vi "Mixed.vi"() -> ()   [LabVIEW 2013]
uses:
  <vilib>/Analysis/4window.llb/windowTd.ctl
  <vilib>/Analysis/NI_AALPro.lvlib
  <vilib>/measure/maspectr.llb/Power Spectrum and PSD Export Mode.ctl
  <vilib>/measure/NI_MAPro.lvlib
  <vilib>/sound2/lvsound2.llb/Sound Output Set Volume (Single).vi
  <vilib>/measure/maspectr.llb/FFT Power Spectrum and PSD for 1 Chan.vi
  <vilib>/measure/maspectr.llb/FFT Spectrum (Mag-Phase) for 1 Chan.vi
  <vilib>/sound2/lvsound2.llb/Sampling Mode.ctl
  <vilib>/sound2/lvsound2.llb/Sound Data Format.ctl
  <vilib>/Analysis/NI_AALBase.lvlib
  <vilib>/sound2/lvsound2.llb/Sound Output Write (DBL Single).vi
panel:
  in  "Triangle":bool
  in  "Random":bool
  in  "Arbitary":bool
  in  "Sine":bool
  in  "Square":bool
  in  "Sawtooth":bool
  in  "Delay (ms)":u32(knob) scale=0.0..1000.0
  in  "STOP":bool
  in  "Frequency Unit":u16(ring) items=["Hz", "cycles"]
  in  "Reset phase":bool
  in  "Sampling rate (Hz)":dbl(knob)=100.0 step=1.0 scale=0.0..100.0
  in  "Frequency (Hz)":dbl(knob)=2.01 step=1.0 scale=0.0..1000.0
  out "Waveform Pattern":dbl[](graph)
  out "Signal Generated":T1(graph)={0.0, 0.01, "arbitrary wave"=[]}
  in  "interpolation":i32(ring)=1 items=["none", "linear"]
  in  "Wave Table":dbl[](array[knob])=[0.0, 1.0, 4.0, 0.2, -0.9] scale=0.0..10.0
  in  "Amplitude":dbl(knob)=3.7755102040816326 scale=0.0..5.0
  in  "Device ID":u32
  in  "Frequency":dbl(knob)=500.0 scale=0.0..10000.0
  out "Generated Sound":waveform(dbl)(graph)
  in  "Volume":dbl(knob)=50.0 scale=0.0..100.0
  out "Y max":dbl format="%0.2f"
  out "Y min":dbl format="%0.2f"
  out "Hz":dbl
  in  "Phase":dbl(knob) scale=0.0..10.0
  out "Power Spectral Density":cluster{"f0":dbl, "df":dbl, "magnitude":dbl[]}(graph)
  out "Magnitude":cluster{"f0":dbl, "df":dbl, "magnitude":dbl[]}(graph)
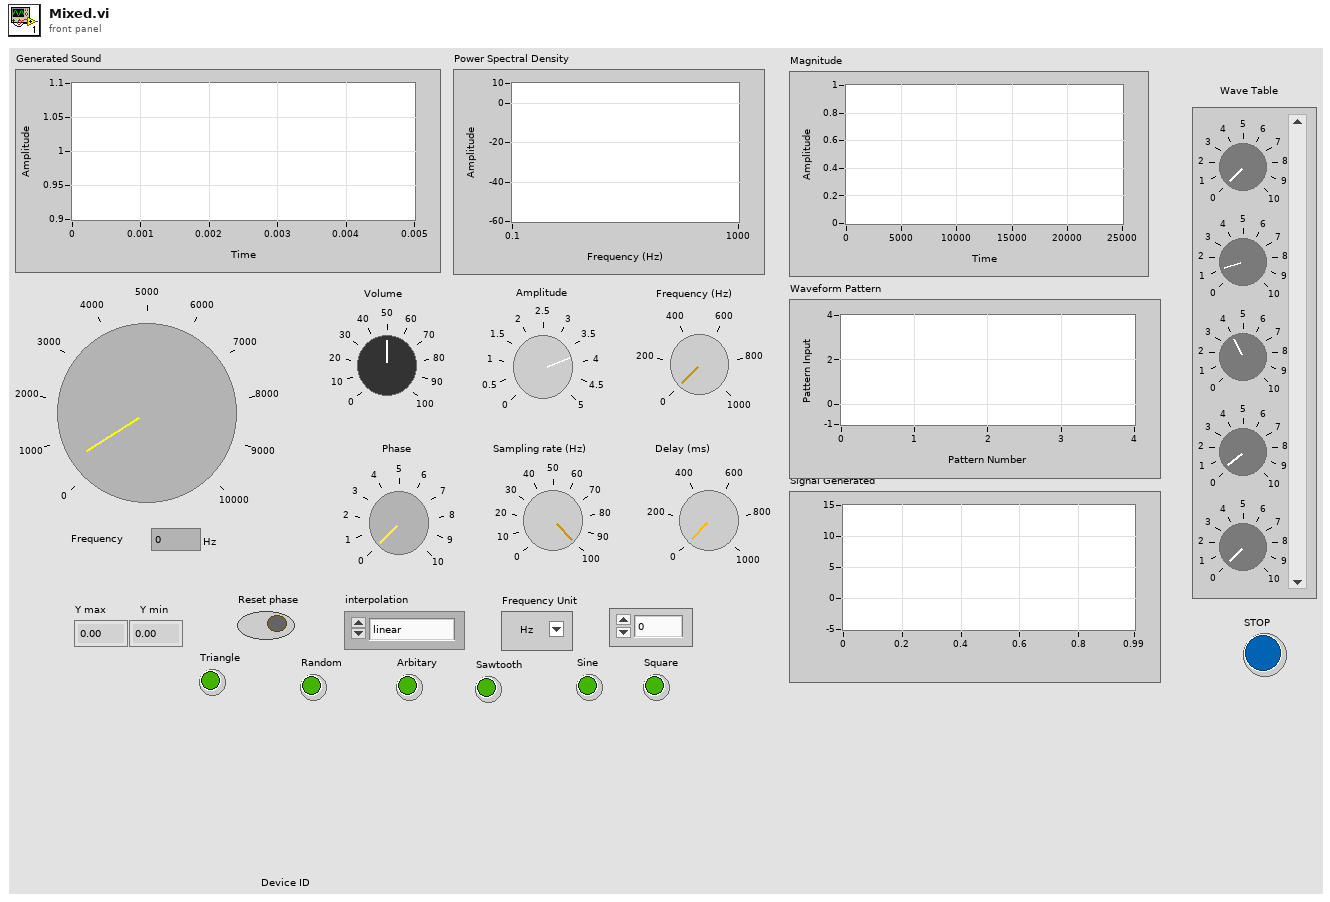
[diagram p1: front panel]
types:
  T1 = cluster{dbl[unit], dbl[unit], "arbitrary wave":dbl[]}
  T2 = typedef "Sound Data Format.ctl" = cluster{"sample rate (S/s)":dbl, "number of channels":i32, "bits per sample":i32}
  T3 = typedef "Sampling Mode.ctl" = i32
  T4 = typedef "Sound Output Task ID.ctl" = u32
  T5 = cluster{"averaging mode":enum16{"No averaging", "Vector averaging", "RMS averaging", "Peak hold"}, "weighting mode":enum16{"Linear", "Exponential"}, "number of averages":u32}
  T6 = cluster{"dB On (F)":bool, "unwrap phase (F)":bool, "convert to degree (F)":bool}
  T7 = typedef "NI_AALPro.lvlib/windowTd.ctl" = u32
  T8 = typedef "NI_MAPro.lvlib/Power Spectrum and PSD Export Mode.ctl" = u16
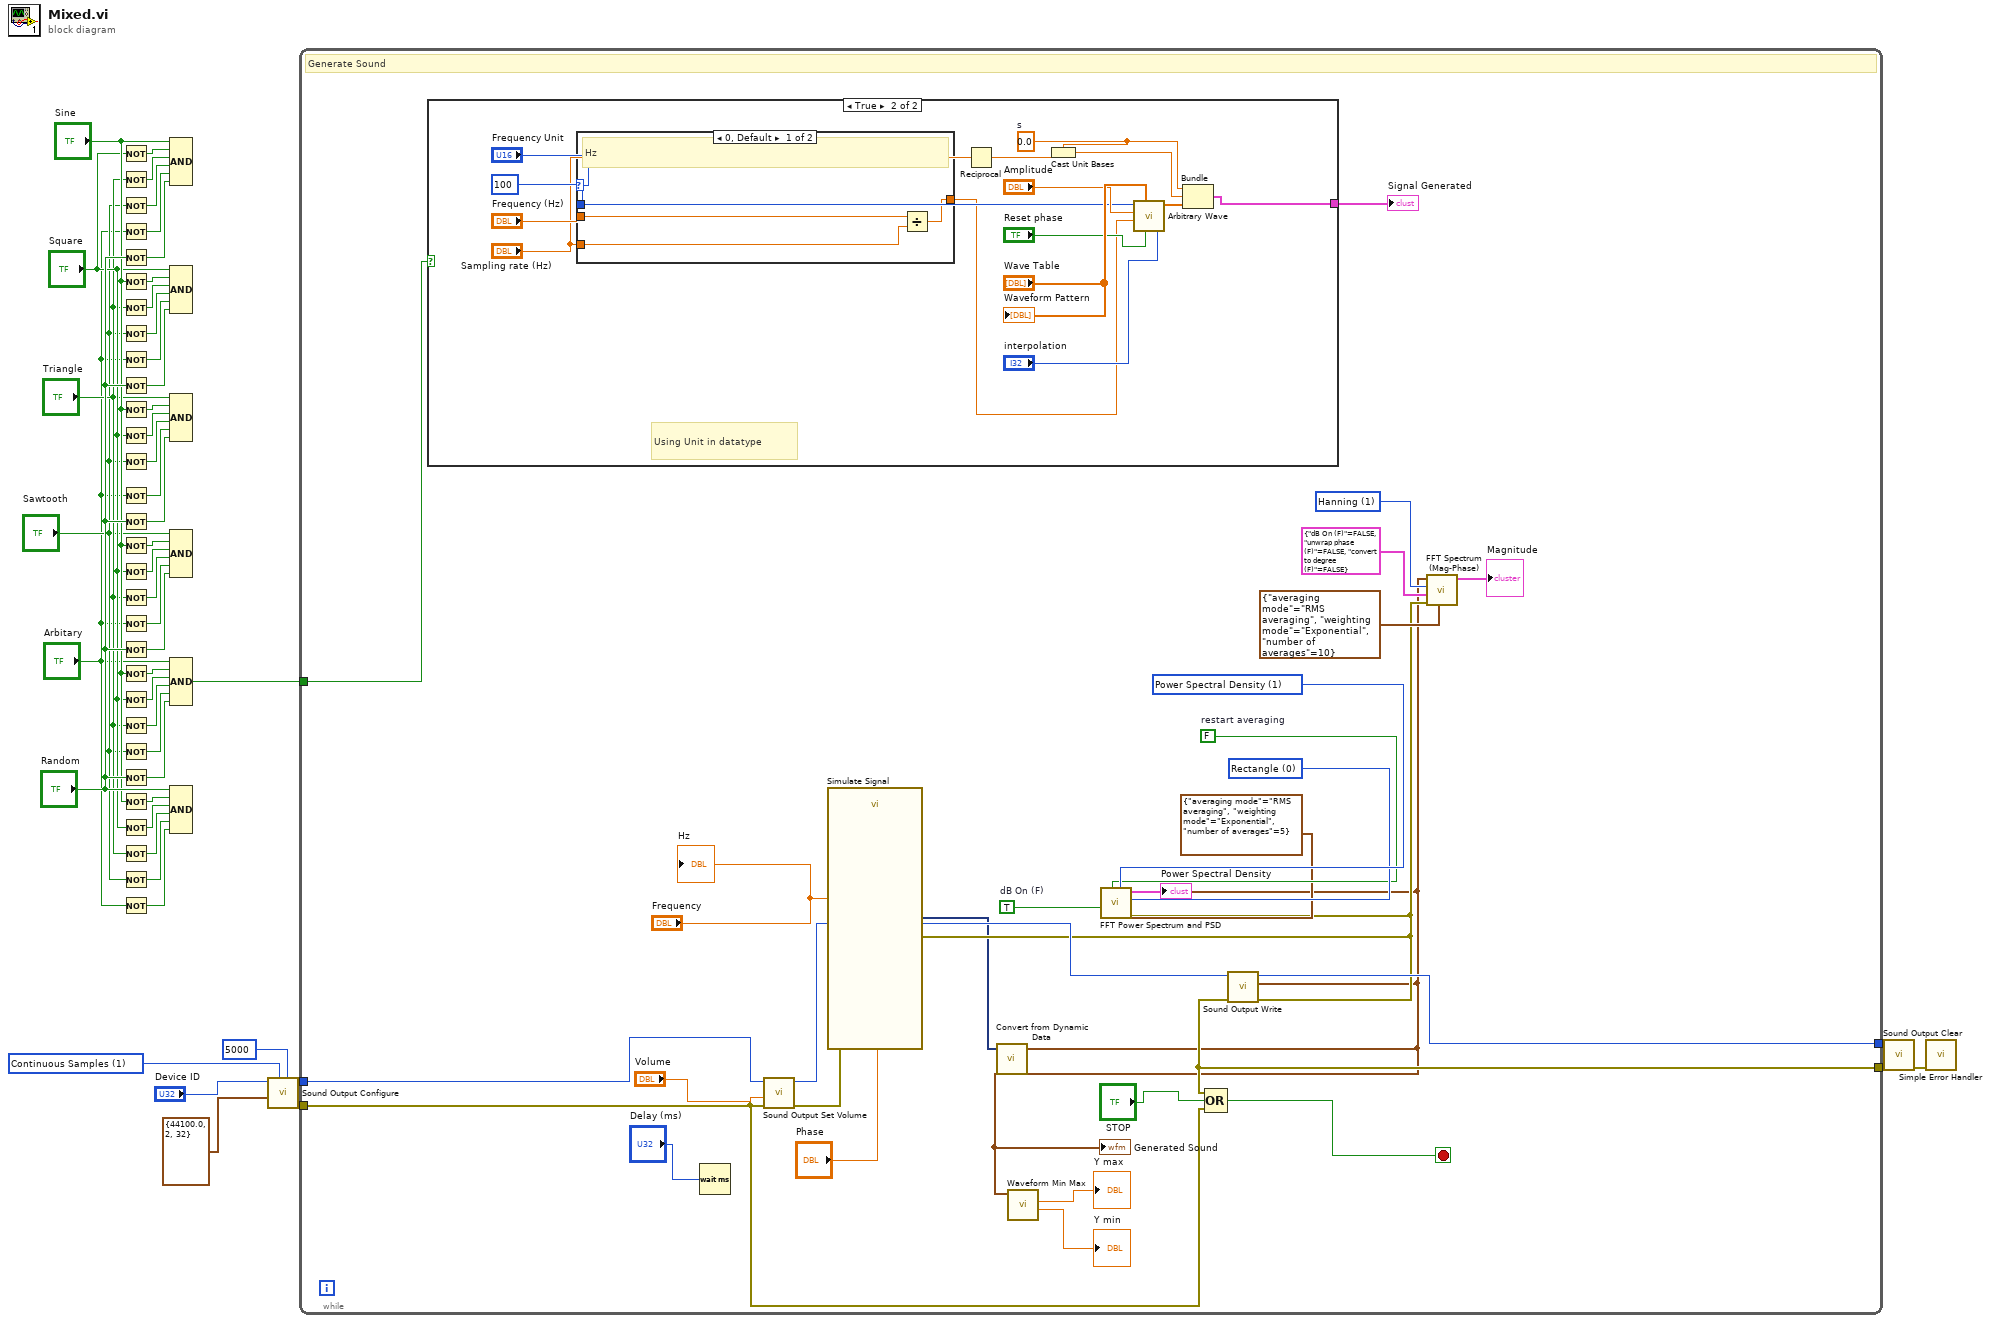
[diagram p0: block diagram]
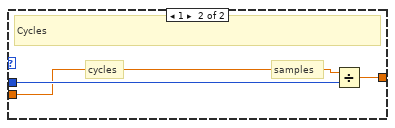
[diagram p3: hidden frame]
diagram:
  w41 = T3 1 items=["Finite Samples", "Continuous Samples"] ("sample mode")
  n1 = Not(x="Square") -> (.not. x?=w37:bool)
  n2 = Not(x="Triangle") -> (.not. x?=w36:bool)
  n3 = Not(x="Sawtooth") -> (.not. x?=w35:bool)
  n4 = Not(x="Arbitary") -> (.not. x?=w34:bool)
  n5 = Not(x="Random") -> (.not. x?=w33:bool)
  n6 = Not(x="Sine") -> (.not. x?=w32:bool)
  n7 = Not(x="Triangle") -> (.not. x?=w31:bool)
  n8 = Not(x="Sawtooth") -> (.not. x?=w30:bool)
  n9 = Not(x="Arbitary") -> (.not. x?=w29:bool)
  n10 = Not(x="Random") -> (.not. x?=w28:bool)
  n11 = Not(x="Sine") -> (.not. x?=w27:bool)
  n12 = Not(x="Square") -> (.not. x?=w26:bool)
  n13 = Not(x="Sawtooth") -> (.not. x?=w25:bool)
  n14 = Not(x="Arbitary") -> (.not. x?=w24:bool)
  n15 = Not(x="Random") -> (.not. x?=w23:bool)
  n16 = Not(x="Sine") -> (.not. x?=w22:bool)
  n17 = Not(x="Square") -> (.not. x?=w21:bool)
  n18 = Not(x="Triangle") -> (.not. x?=w20:bool)
  n19 = Not(x="Arbitary") -> (.not. x?=w19:bool)
  n20 = Not(x="Random") -> (.not. x?=w18:bool)
  n21 = Not(x="Sine") -> (.not. x?=w17:bool)
  n22 = Not(x="Square") -> (.not. x?=w16:bool)
  n23 = Not(x="Triangle") -> (.not. x?=w15:bool)
  n24 = Not(x="Sawtooth") -> (.not. x?=w14:bool)
  n25 = Not(x="Random") -> (.not. x?=w13:bool)
  n26 = Not(x="Sine") -> (.not. x?=w12:bool)
  n27 = Not(x="Square") -> (.not. x?=w11:bool)
  n28 = Not(x="Triangle") -> (.not. x?=w10:bool)
  n29 = Not(x="Sawtooth") -> (.not. x?=w9:bool)
  n30 = Not(x="Arbitary") -> (.not. x?=w8:bool)
  n31 = Compound Arithmetic op=AND("Sine", w37, w36, w35, w34, w33) -> ()  [unwired: 1 out]
  n32 = Compound Arithmetic op=AND("Square", w32, w31, w30, w29, w28) -> ()  [unwired: 1 out]
  n33 = Compound Arithmetic op=AND("Triangle", w27, w26, w25, w24, w23) -> ()  [unwired: 1 out]
  n34 = Compound Arithmetic op=AND("Sawtooth", w22, w21, w20, w19, w18) -> ()  [unwired: 1 out]
  n35 = Compound Arithmetic op=AND("Arbitary", w17, w16, w15, w14, w13) -> (w1:bool)
  n36 = Compound Arithmetic op=AND("Random", w12, w11, w10, w9, w8) -> ()  [unwired: 1 out]
  n37 = call <vilib>:"Sound Output Configure.vi"("number of samples/ch"=5000 ("Number of Samples/ch"), "sample mode"=w41, "sound format"=T2 {"sample rate (S/s)"=44100.0, "number of channels"=2, "bits per sample"=32} ("Sound Format"), "device ID"="Device ID") -> ("error out"=w46:errorcluster, "task ID"=w45:T4)  [unwired: 6 in]
  n38 = while {
    tunnel: w45 -> [w73]
    tunnel: [w75] -> w43
    tunnel: w46 -> [w64]
    tunnel: [w66] -> w44
    tunnel: w1 -> [w48]
    stop <- w65 stop-if-true
    w57 = T7 1 items=["Rectangle"=0, "Hanning"=1, "Hamming"=2, "Blackman-Harris"=3, "Exact Blackman"=4, "Blackman"=5, "Flat Top"=6, "4 Term B-Harris "=7, "7 Term B-Harris"=8, "Low Sidelobe"=9, "Blackman Nuttall"=11, "Triangle"=30, "Bartlett-Hanning"=31, "Bohman"=32, "Parzen"=33, "Welch"=34, "Kaiser"=60, "Dolph-Chebyshev"=61, "Gaussian"=62] ("window")
    w63 = T8 1 items=["Power Spectrum", "Power Spectral Density"] ("export mode")
    w62 = T7 0 items=["Rectangle"=0, "Hanning"=1, "Hamming"=2, "Blackman-Harris"=3, "Exact Blackman"=4, "Blackman"=5, "Flat Top"=6, "4 Term B-Harris "=7, "7 Term B-Harris"=8, "Low Sidelobe"=9, "Blackman Nuttall"=11, "Triangle"=30, "Bartlett-Hanning"=31, "Bohman"=32, "Parzen"=33, "Welch"=34, "Kaiser"=60, "Dolph-Chebyshev"=61, "Gaussian"=62] ("window")
    w60 = FALSE  # restart averaging
    w61 = TRUE  # dB On (F)
    # "Generate Sound"
    n39 = case shown="True" w48 {
      tunnel: [_ w76] -> w47
      frame False {
      }
      frame True {
        w79 = dbl[unit] 0.0  # s
        w87 = 100 ("samples")
        # "Using Unit in datatype"
        n40 = case shown="0, Default" "Frequency Unit" {
          tunnel: [w92 w94] -> w77
          tunnel: w87 -> [_ w95]
          tunnel: "Frequency (Hz)" -> [w91 w93]
          tunnel: "Sampling rate (Hz)" -> [w90 _]
          frame 0, Default {
            # "Hz"
            n41 = Divide(x=w91, y=w90) -> (x/y=w92:dbl)
          }
          frame 1 {
            # "samples"
            # "cycles"
            # "Cycles"
            n42 = Divide(x=w93, y=w95) -> (x/y=w94:dbl)
          }
        }
        n43 = Reciprocal(x="Sampling rate (Hz)") -> (1/x=w82:dbl)
        n44 = Cast Unit Bases(0:w82, 1:w79) -> (2:w81:dbl[unit])
        n45 = call <vilib>:"Arbitrary Wave.vi"("interpolation"="interpolation", "reset phase"="Reset phase", "Wave Table"="Wave Table", "frequency"=w77, "amplitude"="Amplitude", "samples"=w87) -> ("arbitrary wave"=w83:dbl[])  [unwired: 1 in, 2 out]
        n46 = Bundle(w79, w81, "arbitrary wave"=w83) -> (w76:T1)  [unwired: 1 in]
        "Waveform Pattern" <- "Wave Table"
      }
    }
    "Signal Generated" <- w47
    n47 = Wait (ms)(milliseconds to wait="Delay (ms)") -> ()  [unwired: 1 out]
    n48 = call-poly <vilib>:"Sound Output Set Volume.vi"("error in (no error)"=w64, "volume"="Volume", "task ID"=w73) -> ("error out"=w72:errorcluster, "task ID out"=w74:T4)  [unwired: 7 in]
    n49 = call "Simulate Signal"("Frequency"="Frequency", "Phase"="Phase", "error in (no error)"=w72) -> ("Square"=w52:dynamicdata, "error out"=w53:errorcluster)  [unwired: 11 in]
    n50 = call "Convert from Dynamic Data"("Dynamic Data Type"=w52) -> ("Waveform"=w51:waveform(dbl))  [unwired: 3 in]
    "Generated Sound" <- w51
    n51 = call <vilib>:"Waveform Min Max.vi"("waveform in"=w51) -> ("Y min"=→"Y min":dbl, "Y max"=→"Y max":dbl)  [unwired: 5 in, 4 out]
    n52 = call-poly <vilib>:"FFT Power Spectrum and PSD.vi"("export mode"=w63, "averaging parameters"=T5 {"averaging mode"=enum."RMS averaging", "weighting mode"=enum."Exponential", "number of averages"=5}, "restart averaging (F)"=w60, "error in (no error)"=w53, "dB On (F)"=w61, "window"=w62, "time signal"=w51) -> ("Power Spectrum / PSD"=→"Power Spectral Density":cluster{"f0":dbl, "df":dbl, "magnitude":dbl[]})  [unwired: 1 in, 3 out]
    n53 = call-poly <vilib>:"Sound Output Write.vi"("error in (no error)"=w53, "data"=w51, "task ID"=w74) -> ("error out"=w66:errorcluster, "task ID out"=w75:T4)  [unwired: 7 in]
    n54 = Compound Arithmetic op=OR(w66, "STOP", w64) -> (w65:bool)
    n55 = call-poly <vilib>:"FFT Spectrum (Mag-Phase).vi"("averaging parameters"=T5 {"averaging mode"=enum."RMS averaging", "weighting mode"=enum."Exponential", "number of averages"=10}, "error in (no error)"=w53, "view"=T6 {"dB On (F)"=FALSE, "unwrap phase (F)"=FALSE, "convert to degree (F)"=FALSE}, "window"=w57, "time signal"=w51) -> ("magnitude"=→"Magnitude":cluster{"f0":dbl, "df":dbl, "magnitude":dbl[]})  [unwired: 2 in, 4 out]
    "Hz" <- "Frequency"
  }
  n56 = call <vilib>:"Sound Output Clear.vi"("error in (no error)"=w44, "task ID"=w43) -> ("error out"=w39:errorcluster)  [unwired: 9 in]
  n57 = call <vilib>:"Simple Error Handler.vi"("error in (no error)"=w39) -> ()  [unwired: 4 in, 5 out]
